vi "Write To Disk.vi"(8 "error in (no error)":errorcluster, 10 "element":i32[][](array[numeric]), 11 "IntanElectrophysiology in":refnum<class "IntanElectrophysiology.lvclass">) -> (0 "error out":errorcluster, 3 "IntanElectrophysiology out":refnum<class "IntanElectrophysiology.lvclass">)   [LabVIEW 2014, in "IntanElectrophysiology.lvclass"]
uses:
  IntanElectrophysiology.lvclass
  Electrophysiology/Electrophysiology.lvclass
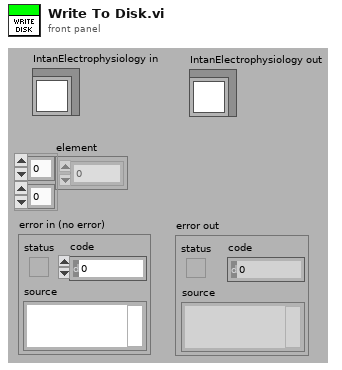
[diagram p1: front panel]
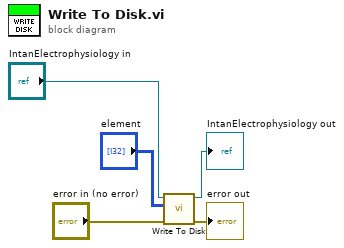
[diagram p0: block diagram]
diagram:
  n1 = call-parent "Write To Disk.vi"("error in (no error)"="error in (no error)", "element"="element", "AcquireTraces in"="IntanElectrophysiology in") -> ("error out"=→"error out":errorcluster, "AcquireTraces out"=→"IntanElectrophysiology out":refnum<class "IntanElectrophysiology.lvclass">)  [unwired: 7 in]
